vi "getInstanceGen.vi"(8 "error in (no error)":errorcluster, 11 "tcpServer in":refnum<class "TcpServer.lvclass">) -> (0 "error out":errorcluster, 2 "GenRead":refnum<user-event>, 3 "tcpServer out":refnum<class "TcpServer.lvclass">)   [LabVIEW 2018, in "TcpServer.lvclass"]
doc: "Get the GenRead user event instance to receive either a generic packet from TCP Client or internal messages, such as errors."
uses:
  TcpServer.lvclass
  TcpServerCmd/typedef/connStatusCluster.ctl
  TcpServer.lvclass/TcpServer.ctl
  TcpServerBase/TcpServerBase.lvclass/TcpServerBase.ctl
  TcpServerCmd/TcpServerCmd.lvclass
  home/pcortes/github/ts_labview_tcp_json/src/TcpServerBase/TcpServerBase.lvclass
  TcpServerBase/TcpServerBase.lvclass
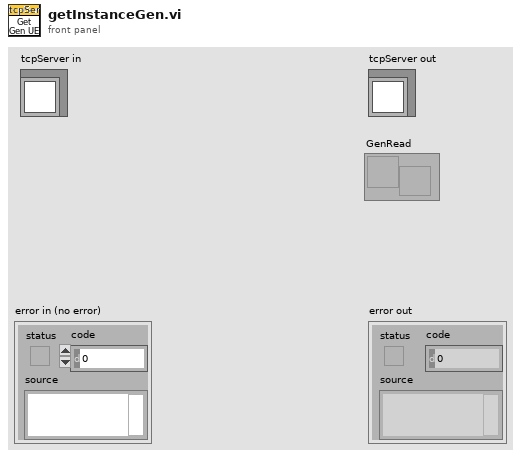
[diagram p1: front panel]
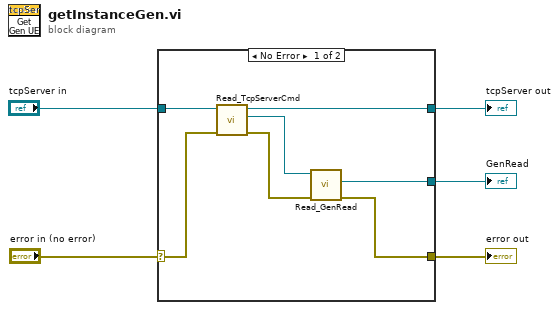
[diagram p0: block diagram]
diagram:
  n1 = case shown="No Error" "error in (no error)" {
    selector: "error in (no error)" -> [w8 w14]
    tunnel: [w6 w14] -> w4
    tunnel: [w11 w13] -> w2
    tunnel: "tcpServer in" -> [w7 w13]
    tunnel: [w9 _] -> w1
    frame No Error {
      n2 = call "Read_TcpServerCmd.vi"("error in (no error)"=w8, "TcpServer in"=w7) -> ("error out"=w12:errorcluster, "TcpServerCmd.lvclass"=w10:refnum<class "TcpServerCmd.lvclass">, "TcpServer out"=w11:refnum<class "TcpServer.lvclass">)  [unwired: 7 in]
      n3 = call "Read_GenRead.vi"("error in (no error)"=w12, "TcpServerBase in"=w10) -> ("error out"=w6:errorcluster, "GenRead"=w9:refnum<user-event>)  [unwired: 7 in, 1 out]
    }
    frame Error {
    }
  }
  "error out" <- w4
  "tcpServer out" <- w2
  "GenRead" <- w1
